vi "Error Bar Page.vi"() -> ()   [LabVIEW 2017, in "2D Error Bar.lvclass"]
uses:
  <vilib>/Math Plots/2D Math Plots/2D Error Bar/2D Error Bar/2D Error Bar.lvclass
  <vilib>/Math Plots/2D Math Plots/2D Plot/Action String/2DMathPlot Ctrl Act Queue.ctl
  <vilib>/Math Plots/2D Math Plots/2D Plot/Action String/2DMathPlot Ctrl Act Cluster.ctl
  <vilib>/Math Plots/2D Math Plots/2D Plot/Action String/2DMathPlot State Class.ctl
  <vilib>/Math Plots/2D Math Plots/2D Error Bar/2D Error Bar/Typedef/2D Error Bar Property Cluster.ctl
  <vilib>/Math Plots/2D Math Plots/2D Plot/2D Plot/Typedef/Plot Property Array.ctl
  <vilib>/Math Plots/2D Math Plots/2D Plot/2D Plot/Typedef/Plot Property.ctl
  <vilib>/Math Plots/2D Math Plots/2D Error Bar/2D Error Bar/Typedef/2D Error Bar Property Array.ctl
  <vilib>/Math Plots/2D Math Plots/2D Error Bar/2D Error Bar/Typedef/2D Error Bar Property.ctl
  <vilib>/Math Plots/2D Math Plots/2D Plot/2D Plot/Typedef/Dialog State.ctl
  <vilib>/Math Plots/2D Math Plots/2D Plot/2D Plot/Typedef/Temp Graph State.ctl
  <vilib>/Math Plots/2D Math Plots/2D Plot/2D Plot/Typedef/Temp Graph Property Action.ctl
  <vilib>/Math Plots/2D Math Plots/2D Plot/2D Plot/2D Plot.lvclass
panel:
  in  "Fill to":i32(ring)=-1 items=["<none>"=-1, "zero"=-2, "-Infinity"=-3, "+Infinity"=-4, "-"=100]
  in  "Errorbar Point/fill":u32(colorbox)=16777215 caption="Point/fill color"
  in  "Errorbar Interpolation":T1
  in  "Errorbar Line Width":T2
  in  "Errorbar Point Style":T3
  in  "Errorbar Line Style":T4
  in  "Errorbar Line Color":u32(colorbox) caption="Line color"
  in  "Error Mode":u16(ring) items=["Y errorbar", "XY errorbar"]
  in  "Marker Color":u32(colorbox) caption="Marker color"
  out "Error Bar Property Out":T5={"Plot Property Array"=[{"Bar Plot Style"=0, "DigitalLineStyle"=1, "TransitionLocation"=0, "Transition Type"=0, "Fill To"=0, "Fill/Pt. Color"=0, "Label Style"=0, "Line Style"=0, "Line Width"=0, "Plot Color"=0, "Plot Interpolation"=0, "Plot Name"="", "Point Style"=0, "Visible?"=FALSE, "XScaleIdx"=0, "YScaleIdx"=0}, {"Bar Plot Style"=0, "DigitalLineStyle"=1, "TransitionLocation"=0, "Transition Type"=0, "Fill To"=0, "Fill/Pt. Color"=0, "Label Style"=0, "Line Style"=0, "Line Width"=0, "Plot Color"=0, "Plot Interpolation"=0, "Plot Name"="", "Point Style"=0, "Visible?"=FALSE, "XScaleIdx"=0, "YScaleIdx"=0}], "2D Error Bar Property Array"=[]}
  in  "Error Bar Property In":T5={"Plot Property Array"=[{"Bar Plot Style"=0, "DigitalLineStyle"=1, "TransitionLocation"=0, "Transition Type"=0, "Fill To"=0, "Fill/Pt. Color"=0, "Label Style"=0, "Line Style"=0, "Line Width"=0, "Plot Color"=0, "Plot Interpolation"=0, "Plot Name"="", "Point Style"=0, "Visible?"=FALSE, "XScaleIdx"=0, "YScaleIdx"=0}, {"Bar Plot Style"=0, "DigitalLineStyle"=1, "TransitionLocation"=0, "Transition Type"=0, "Fill To"=0, "Fill/Pt. Color"=0, "Label Style"=0, "Line Style"=0, "Line Width"=0, "Plot Color"=0, "Plot Interpolation"=0, "Plot Name"="", "Point Style"=0, "Visible?"=FALSE, "XScaleIdx"=0, "YScaleIdx"=0}], "2D Error Bar Property Array"=[]}
  in  "Event Registration":refnum<event-registration>
  in  "Control Ref Queue":T10
  in  "Marker Size":dbl=0.001 caption="Size" min=0.001 step=1.0
  in  "Marker Line Width":T2
  in  "Marker Line Style":T4
  in  "Name":string
  in  "Active Plot":i32(ring) items=["Plot 0"]
  # "Error Bar"
  # "Error Marker"
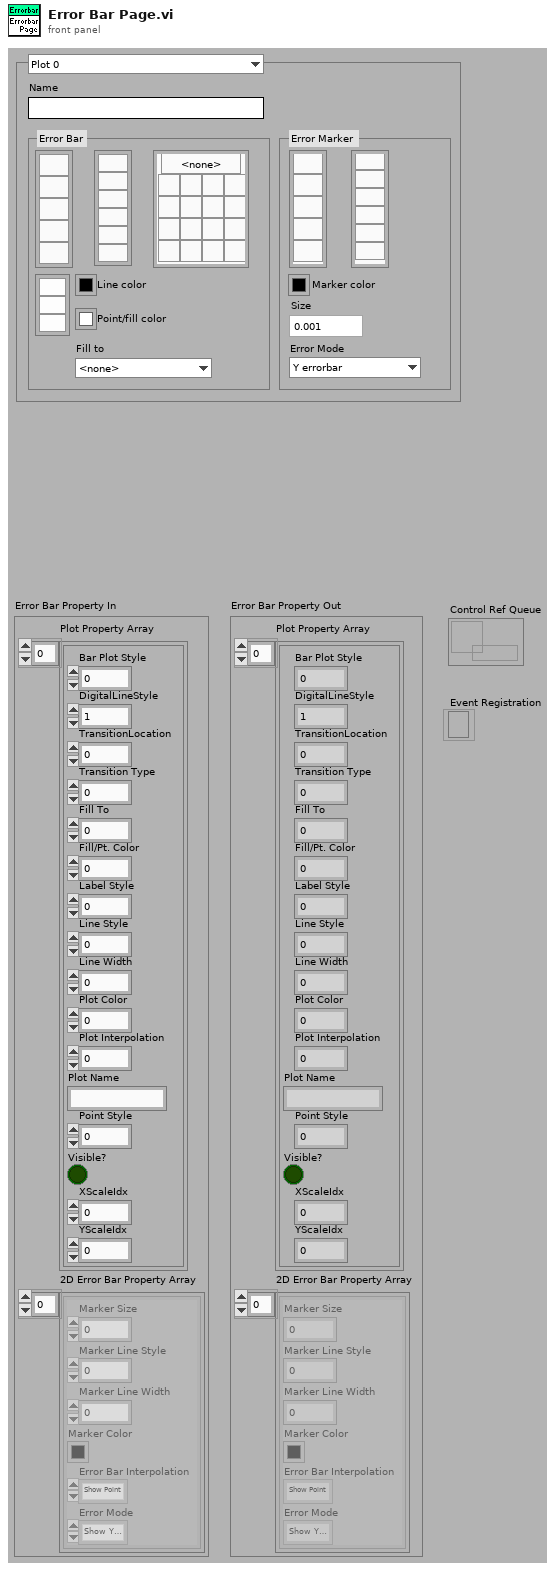
[diagram p1: front panel]
types:
  T1 = cluster{"OK Button 2":bool, "OK Button 4":bool, "OK Button 6":bool}
  T2 = cluster{"OK Button 2":bool, "OK Button 3":bool, "OK Button 4":bool, "OK Button 5":bool, "OK Button 6":bool, "OK Button 7":bool}
  T3 = cluster{"OK Button 17":bool, "OK Button":bool, "OK Button 2":bool, "OK Button 3":bool, "OK Button 4":bool, "OK Button 5":bool, "OK Button 6":bool, "OK Button 7":bool, "OK Button 8":bool, "OK Button 9":bool, "OK Button 10":bool, "OK Button 11":bool, "OK Button 12":bool, "OK Button 13":bool, "OK Button 14":bool, "OK Button 15":bool, "OK Button 16":bool}
  T4 = cluster{"OK Button":bool, "OK Button 2":bool, "OK Button 3":bool, "OK Button 4":bool, "OK Button 5":bool}
  T5 = typedef "2D Error Bar.lvclass/2D Error Bar Property Cluster.ctl" = cluster{"Plot Property Array":T6, "2D Error Bar Property Array":T8}
  T6 = typedef "2D Plot.lvclass/Plot Property Array.ctl" = T7[]
  T7 = typedef "2D Plot.lvclass/Plot Property.ctl" = cluster{"Bar Plot Style":u8, "DigitalLineStyle":u8, "TransitionLocation":u8, "Transition Type":u8, "Fill To":i16, "Fill/Pt. Color":u32, "Label Style":u8, "Line Style":u8, "Line Width":u8, "Plot Color":u32, "Plot Interpolation":u8, "Plot Name":string, "Point Style":u8, "Visible?":bool, "XScaleIdx":u32, "YScaleIdx":u32}
  T8 = typedef "2D Error Bar.lvclass/2D Error Bar Property Array.ctl" = T9[]
  T9 = typedef "2D Error Bar.lvclass/2D Error Bar Property.ctl" = cluster{"Marker Size":dbl, "Marker Line Style":u8, "Marker Line Width":u8, "Marker Color":u32, "Error Bar Interpolation":enum16{"Show Point", "Show Line", "Show Bar"}, "Error Mode":enum16{"Show Y Error", "Show X Error", "Show Both Error"}}
  T10 = typedef "2DMathPlot Ctrl Act Queue.ctl" = refnum<queue>
  T11 = typedef "2D Plot.lvclass/Dialog State.ctl" = enum16{"Initialize", "Read Property", "Write Property", "Idle", "Exit"}
  T12 = typedef "2DMathPlot Ctrl Act Cluster.ctl" = cluster{"Plot Area Ref":refnum<vi>, "Z Axis Ref":refnum<vi>, "Legend Ref":refnum<vi>, "XControl Ref":refnum<vi>, "Facade Ref":refnum<vi>, "Display State Change Class":T13}
  T13 = typedef "2DMathPlot State Class.ctl" = enum16{"Update All (Undo)", "Update General", "Update Appearance", "Update Format", "Update Scale", "Update Marker", "Update Cursor", "None"}
  T14 = typedef "2D Plot.lvclass/Temp Graph Property Action.ctl" = enum16{"Appearance Property", "Format Property", "Plots Property", "Scales Property"}
  T15 = typedef "2D Plot.lvclass/Temp Graph State.ctl" = enum16{"Create", "Update Graph", "Update Property Only", "Get Plot Name", "Get Axis Name", "Destory"}
  T16 = enum16{"Show Y Error", "Show X Error", "Show Both Error"}
  T17 = cluster{"Bool Array[0]":bool, "Bool Array[1]":bool, "Bool Array[2]":bool, "Bool Array[3]":bool, "Bool Array[4]":bool}
  T18 = cluster{"Bool Array[0]":bool, "Bool Array[1]":bool, "Bool Array[2]":bool, "Bool Array[3]":bool, "Bool Array[4]":bool, "Bool Array[5]":bool}
  T19 = cluster{"Bool Array[0]":bool, "Bool Array[1]":bool, "Bool Array[2]":bool, "Bool Array[3]":bool, "Bool Array[4]":bool, "Bool Array[5]":bool, "Bool Array[6]":bool, "Bool Array[7]":bool, "Bool Array[8]":bool, "Bool Array[9]":bool, "Bool Array[10]":bool, "Bool Array[11]":bool, "Bool Array[12]":bool, "Bool Array[13]":bool, "Bool Array[14]":bool, "Bool Array[15]":bool, "Bool Array[16]":bool}
  T20 = cluster{"Bool Array[0]":bool, "Bool Array[1]":bool, "Bool Array[2]":bool}
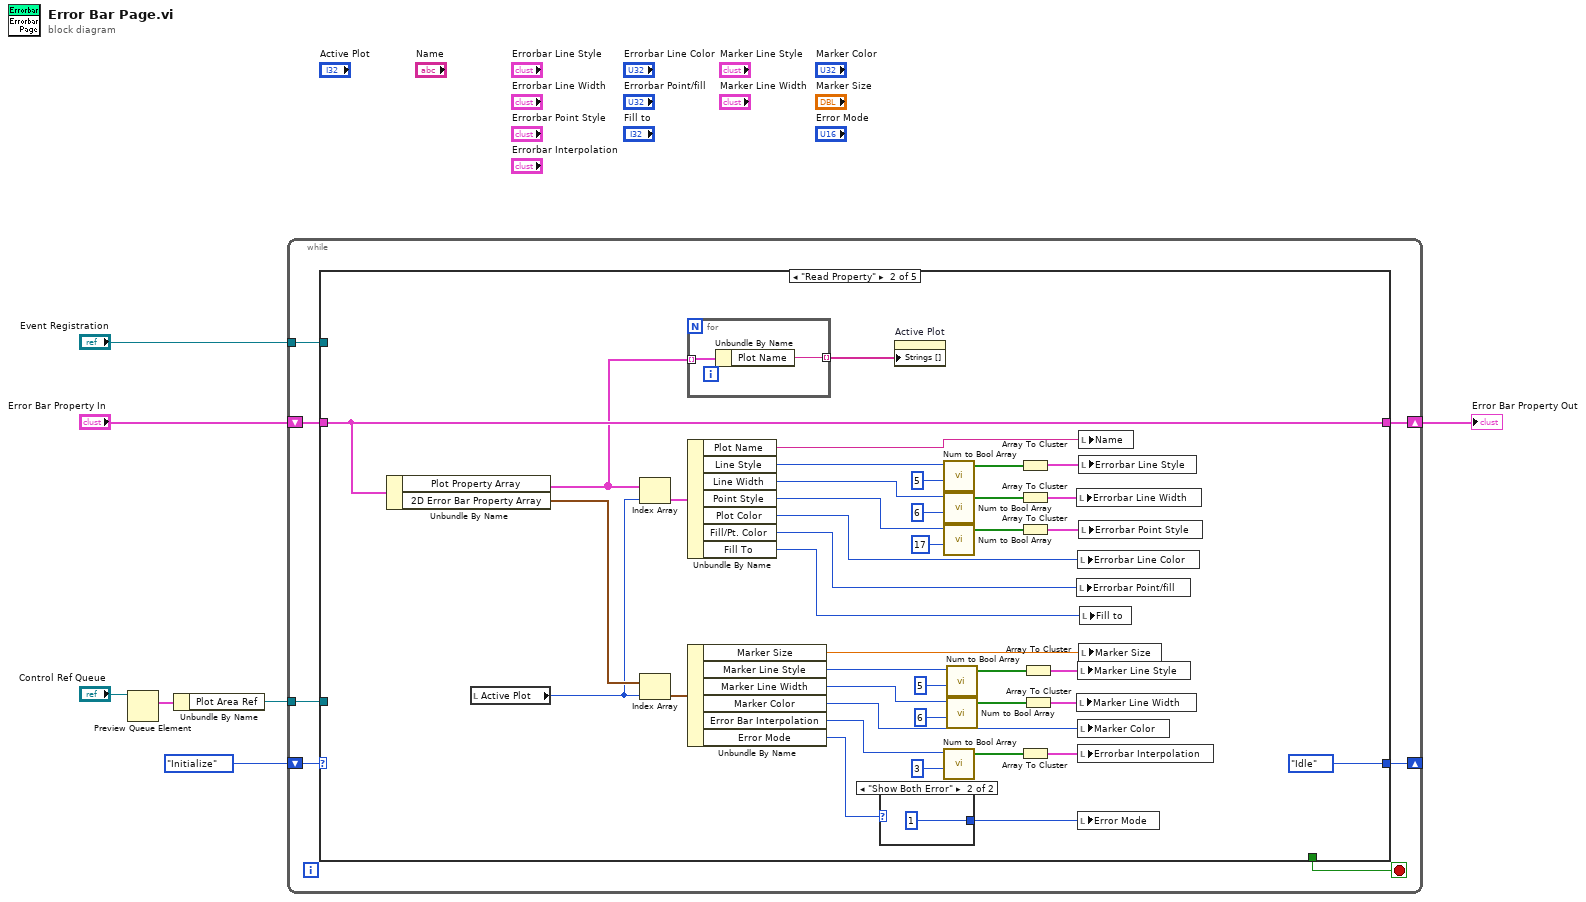
[diagram p0: block diagram]
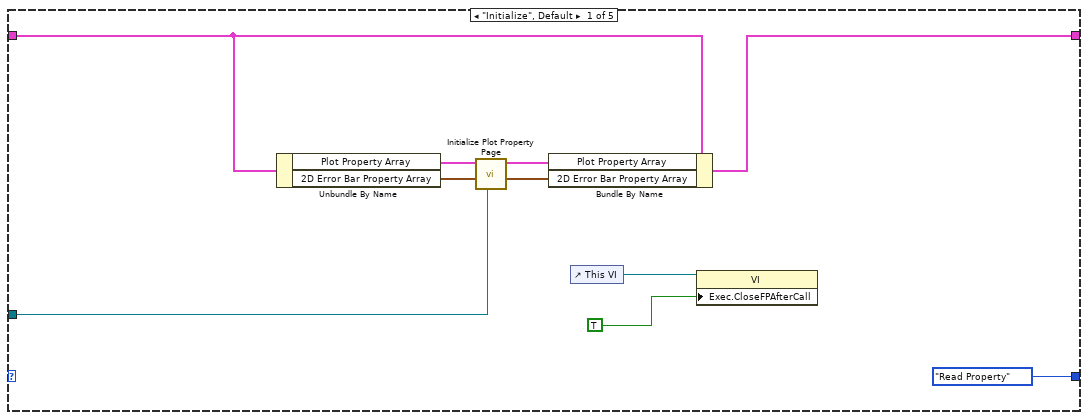
[diagram p2: hidden frame]
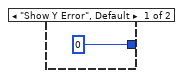
[diagram p3: hidden frame]
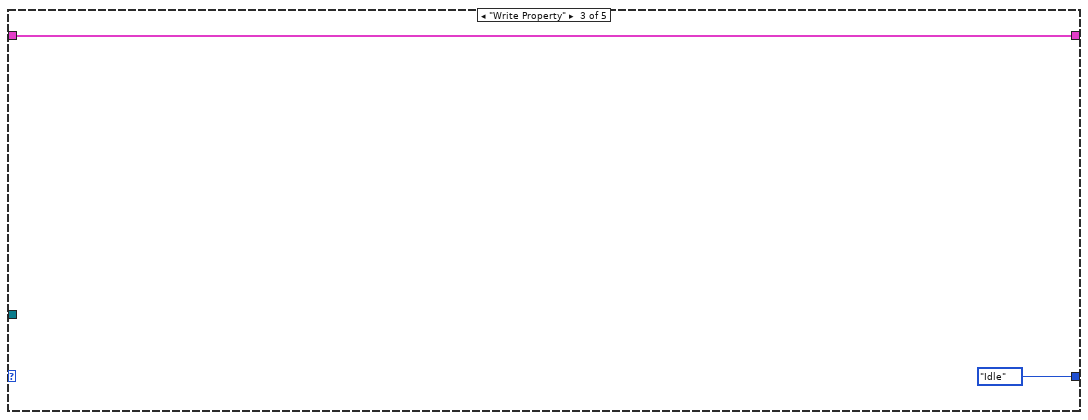
[diagram p4: hidden frame]
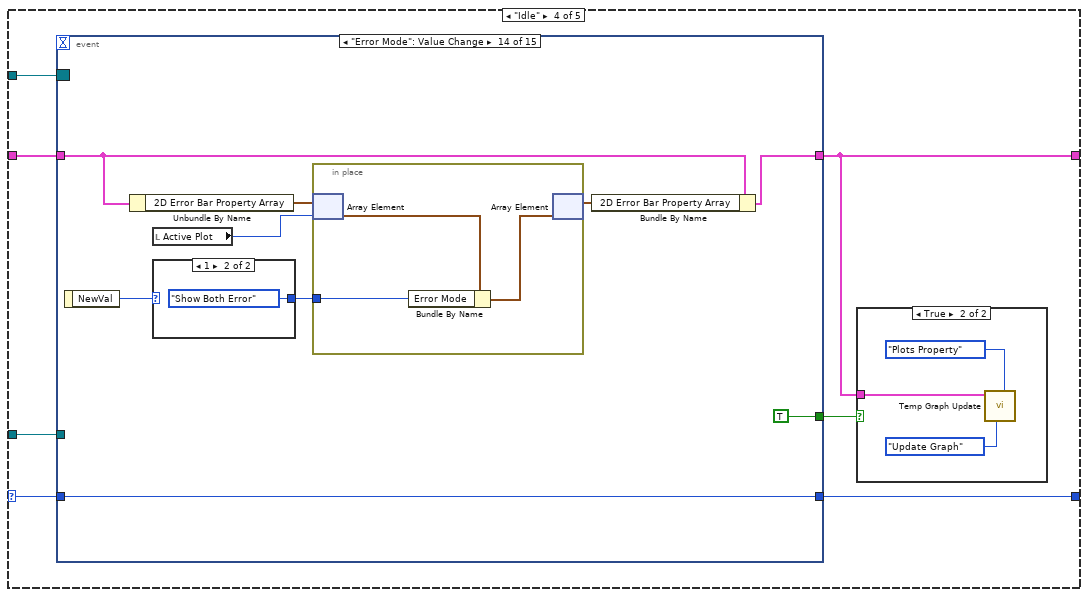
[diagram p5: hidden frame]
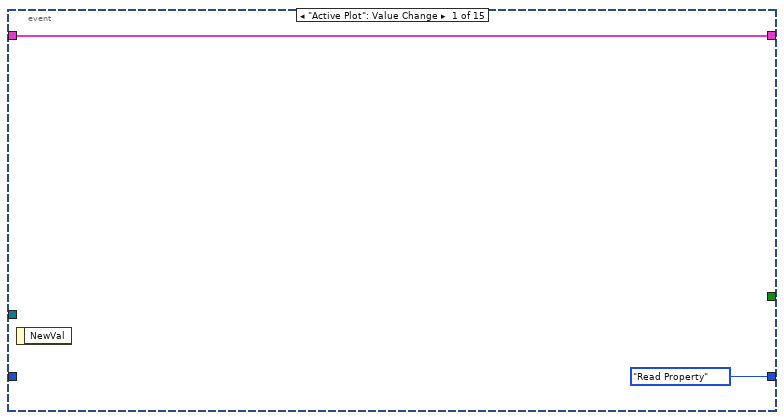
[diagram p7: hidden frame]
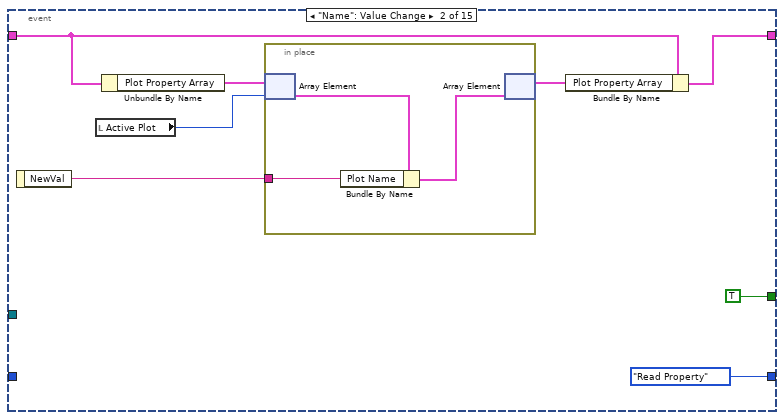
[diagram p8: hidden frame]
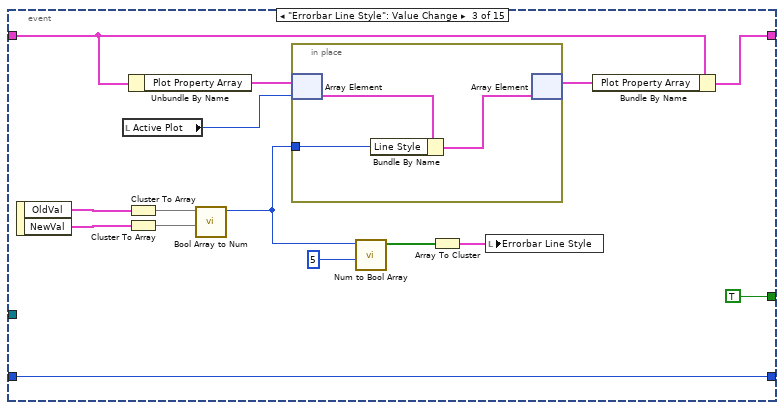
[diagram p9: hidden frame]
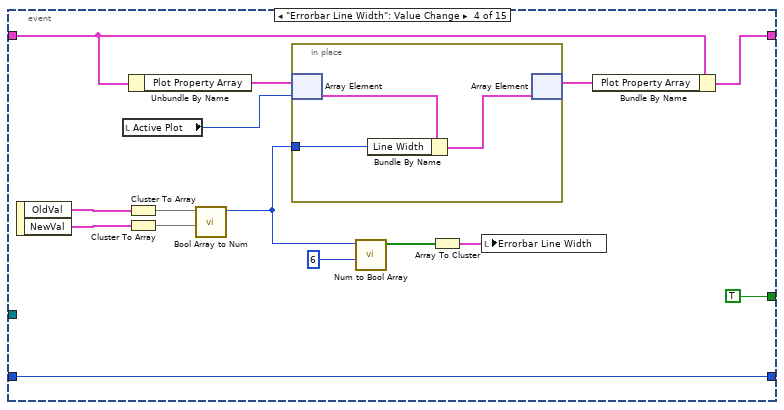
[diagram p10: hidden frame]
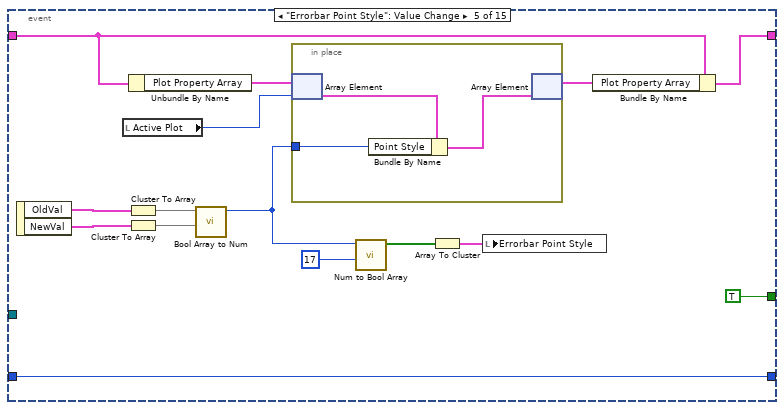
[diagram p11: hidden frame]
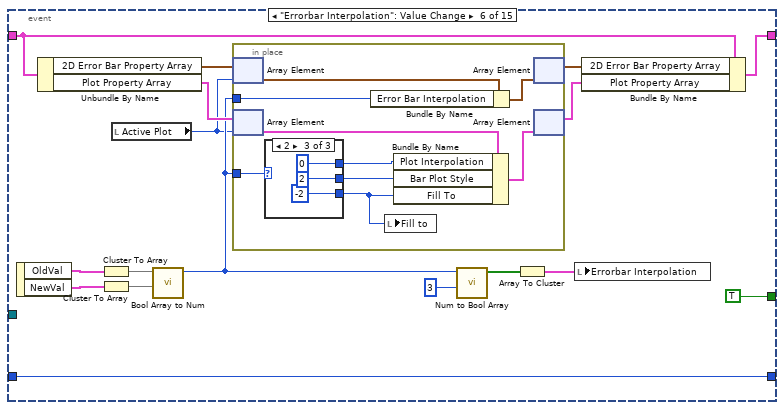
[diagram p12: hidden frame]
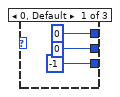
[diagram p13: hidden frame]
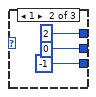
[diagram p14: hidden frame]
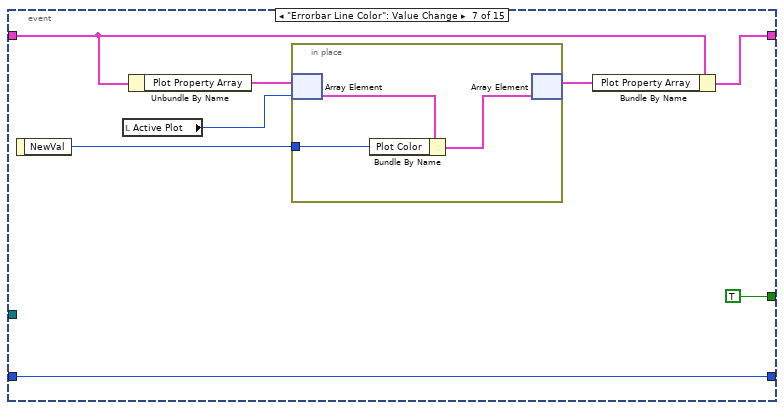
[diagram p15: hidden frame]
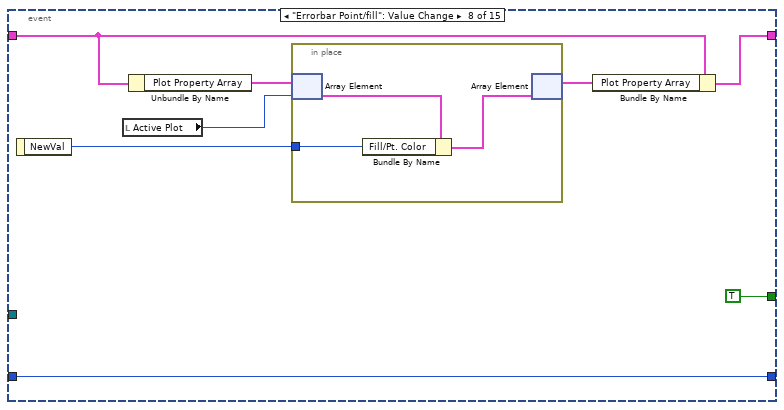
[diagram p16: hidden frame]
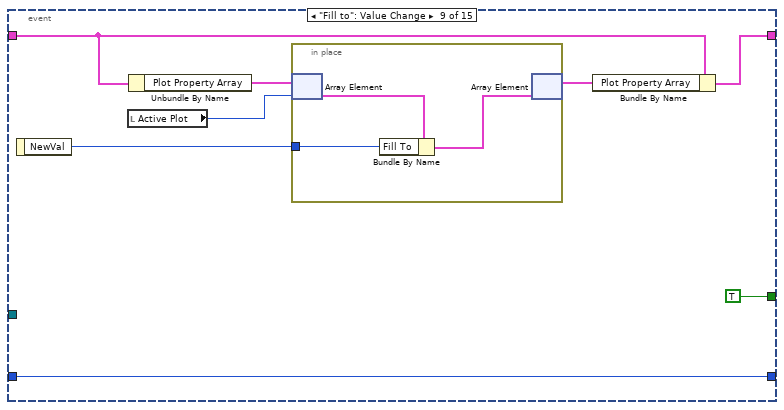
[diagram p17: hidden frame]
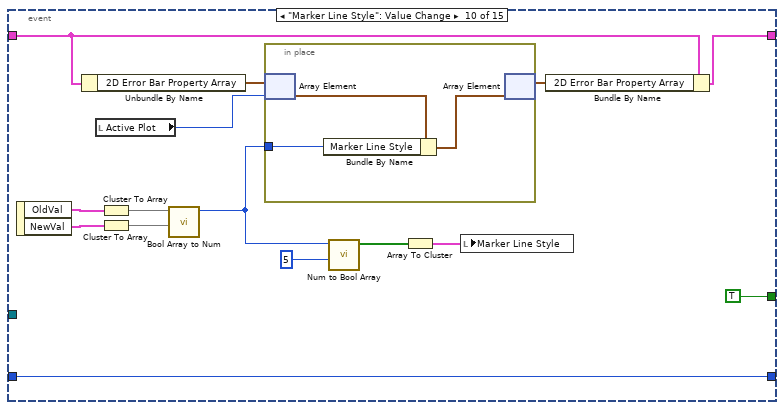
[diagram p18: hidden frame]
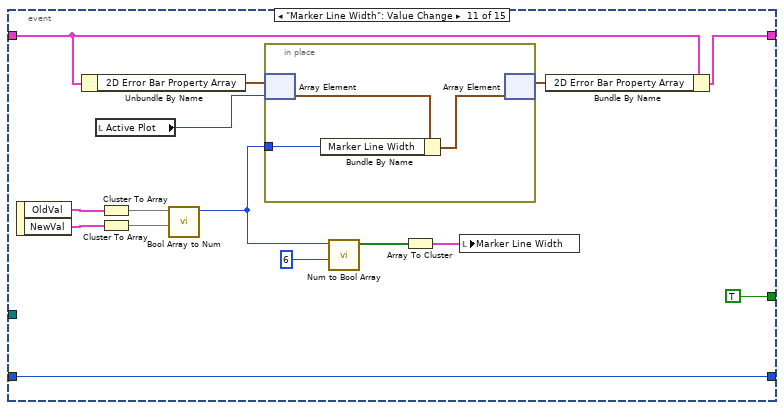
[diagram p19: hidden frame]
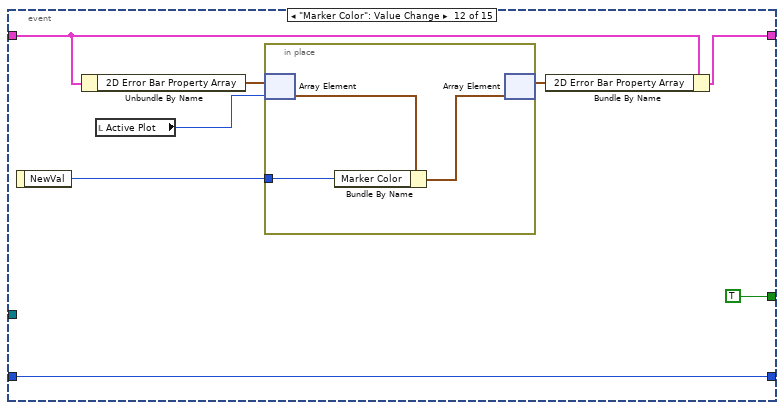
[diagram p20: hidden frame]
diagram:
  n1 = Preview Queue Element(queue="Control Ref Queue") -> (element=w5:T12)  [unwired: 1 in, 4 out]
  n2 = Unbundle By Name(w5) -> ("Plot Area Ref"=w4:refnum<vi>)
  n3 = while {
    tunnel: w4 -> [w13]
    tunnel: "Event Registration" -> [w12]
    shift-right: [w9] -> _
    shift-left: Dialog_State."Initialize" ("Enum") -> [w14]
    shift-right: [w10] -> w1
    shift-left: "Error Bar Property In" -> [w11]
    stop <- w8 stop-if-true
    n4 = case shown="\"Read Property\"" w14 {
      selector: w14 -> [_ _ _ w74 w292]
      tunnel: w13 -> [w15 _ _ w75 _]
      tunnel: w12 -> [_ _ _ w77 _]
      tunnel: w11 -> [w21 w61 w69 w76 w290]
      tunnel: [w20 w61 w69 w73 w290] -> w10
      tunnel: [Dialog_State."Read Property" ("Enum") Dialog_State."Idle" ("Enum") Dialog_State."Idle" ("Enum") w72 w292] -> w9
      tunnel: [_ _ _ _ TRUE] -> w8
      frame "Initialize", Default {
        n5 = Unbundle By Name(w21) -> ("Plot Property Array"=w19:T6, "2D Error Bar Property Array"=w18:T8)
        n6 = call <vilib>:"Initialize Plot Property Page.vi"("Plot Area Ref"=w15, "2D Error Bar Array In"=w18, "Plot Property Array In"=w19) -> ("2D Error Bar Array Out"=w16:T8, "Plot Property Array Out"=w17:T6)  [unwired: 2 in, 5 out]
        n7 = Bundle By Name(cluster=w21, "Plot Property Array"=w17, "2D Error Bar Property Array"=w16) -> (w20:T5)
        n8 = control-ref of="This VI"() -> (w23:refnum<vi>)
        n9 = property class="VI"(reference=w23, "Exec.CloseFPAfterCall"=TRUE ("Execution:Close After Call")) -> ()  [unwired: 1 in, 2 out]
      }
      frame "Read Property" {
        n10 = Unbundle By Name(w61) -> ("Plot Property Array"=w49:T6, "2D Error Bar Property Array"=w64:T8)
        n11 = local read "Active Plot"() -> (w28:i32)
        n12 = Index Array(array=w49, index=w28) -> (element=w63:T7)
        n13 = Index Array(array=w64, index=w28) -> (element=w62:T9)
        n14 = for {
          tunnel: w49 -> [w68] mode=indexing
          tunnel: [w67] -> w48 mode=indexing
          n15 = Unbundle By Name(w68) -> ("Plot Name"=w67:string)
        }
        n16 = Unbundle By Name(w63) -> ("Plot Name"=w59:string, "Line Style"=w58:u8, "Line Width"=w51:u8, "Point Style"=w35:u8, "Plot Color"=w32:u32, "Fill/Pt. Color"=w31:u32, "Fill To"=w30:i16)
        n17 = Unbundle By Name(w62) -> ("Marker Size"=w60:dbl, "Marker Line Style"=w43:u8, "Marker Line Width"=w41:u8, "Marker Color"=w25:u32, "Error Bar Interpolation"=w29:enum16{"Show Point", "Show Line", "Show Bar"}, "Error Mode"=w27:T16)
        n18 = case shown="\"Show Both Error\"" w27 {
          tunnel: [0 1] -> w26
          frame "Show Y Error", Default {
          }
          frame "Show Both Error" {
          }
        }
        n19 = property on="Active Plot" class="Ring (strict)"("Strings []"=w48) -> ()  [unwired: 2 in, 2 out]
        n20 = call <vilib>:"Num to Bool Array.vi"("Array Size"=5, "Value"=w58) -> ("Bool Array"=w56:bool[])  [unwired: 9 out]
        n21 = call <vilib>:"Num to Bool Array.vi"("Array Size"=6, "Value"=w51) -> ("Bool Array"=w54:bool[])  [unwired: 9 out]
        n22 = call <vilib>:"Num to Bool Array.vi"("Array Size"=17, "Value"=w35) -> ("Bool Array"=w37:bool[])  [unwired: 9 out]
        n23 = call <vilib>:"Num to Bool Array.vi"("Array Size"=3, "Value"=w29) -> ("Bool Array"=w39:bool[])  [unwired: 9 out]
        n24 = call <vilib>:"Num to Bool Array.vi"("Array Size"=5, "Value"=w43) -> ("Bool Array"=w45:bool[])  [unwired: 9 out]
        n25 = call <vilib>:"Num to Bool Array.vi"("Array Size"=6, "Value"=w41) -> ("Bool Array"=w46:bool[])  [unwired: 9 out]
        n26 = Array To Cluster(array=w56) -> (cluster=w55:T17)
        n27 = Array To Cluster(array=w54) -> (cluster=w52:T18)
        n28 = Array To Cluster(array=w37) -> (cluster=w33:T19)
        n29 = Array To Cluster(array=w39) -> (cluster=w34:T20)
        n30 = Array To Cluster(array=w45) -> (cluster=w42:T17)
        n31 = Array To Cluster(array=w46) -> (cluster=w40:T18)
        n32 = local write "Errorbar Line Width"(w52) -> ()
        n33 = local write "Errorbar Point/fill"(w31) -> ()
        n34 = local write "Marker Line Width"(w40) -> ()
        n35 = local write "Errorbar Line Color"(w32) -> ()
        n36 = local write "Marker Line Style"(w42) -> ()
        n37 = local write "Marker Color"(w25) -> ()
        n38 = local write "Errorbar Interpolation"(w34) -> ()
        n39 = local write "Error Mode"(w26) -> ()
        n40 = local write "Name"(w59) -> ()
        n41 = local write "Errorbar Line Style"(w55) -> ()
        n42 = local write "Errorbar Point Style"(w33) -> ()
        n43 = local write "Marker Size"(w60) -> ()
        n44 = local write "Fill to"(w30) -> ()
      }
      frame "Write Property" {
      }
      frame "Idle" {
        n45 = event shown="[13] \"Error Mode\": Value Change" {
          selector: w77 -> [_ _ _ _ _ _ _ _ _ _ _ _ _ _ _]
          dyn-events: _ -> [_ _ _ _ _ _ _ _ _ _ _ _ _ _ _]
          timeout: _ -> [_ _ _ _ _ _ _ _ _ _ _ _ _ _ _]
          tunnel: w76 -> [w82 w90 w100 w118 w136 w157 w187 w198 w209 w230 w248 w259 w270 w282 w288]
          tunnel: w75 -> [_ _ _ _ _ _ _ _ _ _ _ _ _ _ _]
          tunnel: [w82 w89 w99 w117 w135 w156 w186 w197 w208 w229 w247 w258 w269 w281 w288] -> w73
          tunnel: [Dialog_State."Read Property" ("Enum") Dialog_State."Read Property" ("Enum") w96 w114 w132 w153 w185 w196 w207 w218 w235 w254 w265 w277 Dialog_State."Exit" ("Enum")] -> w72
          tunnel: w74 -> [_ _ w96 w114 w132 w153 w185 w196 w207 w218 w235 w254 w265 w277 _]
          tunnel: [_ TRUE TRUE TRUE TRUE TRUE TRUE TRUE TRUE TRUE TRUE TRUE TRUE TRUE _] -> w71
          event "Active Plot": Value Change {
            n46 = event-data() -> ()  [unwired: 2 out]
          }
          event "Name": Value Change {
            n47 = event-data() -> ("NewVal"=w85:string)  [unwired: 1 out]
            n48 = local read "Active Plot"() -> (w87:i32)
            n49 = Unbundle By Name(w90) -> ("Plot Property Array"=w88:T6)
            n50 = in-place {
              in-place-border: w85 -> [w91]
              n51 = in-place-array #1(w88, w87) -> (w93:T7)
              n52 = Bundle By Name(cluster=w93, "Plot Name"=w91) -> (w92:T7)
              n53 = in-place-array #1(w92) -> (w86:T6)  [unwired: 1 out]
            }
            n54 = Bundle By Name(cluster=w90, "Plot Property Array"=w86) -> (w89:T5)
          }
          event "Errorbar Line Style": Value Change {
            n55 = event-data() -> ("OldVal"=w98:T4, "NewVal"=w97:T4)  [unwired: 1 out]
            n56 = local read "Active Plot"() -> (w101:i32)
            n57 = Cluster To Array(cluster=w98) -> (array=w104:bool[])
            n58 = Cluster To Array(cluster=w97) -> (array=w103:bool[])
            n59 = Unbundle By Name(w100) -> ("Plot Property Array"=w108:T6)
            n60 = call <vilib>:"Bool Array to Num.vi"("New Bool Array"=w103, "Old Bool Array"=w104) -> ("Value"=w95:u8)  [unwired: 9 out]
            n61 = in-place {
              in-place-border: w95 -> [w109]
              n62 = in-place-array #2(w108, w101) -> (w111:T7)
              n63 = Bundle By Name(cluster=w111, "Line Style"=w109) -> (w110:T7)
              n64 = in-place-array #2(w110) -> (w107:T6)  [unwired: 1 out]
            }
            n65 = call <vilib>:"Num to Bool Array.vi"("Array Size"=5, "Value"=w95) -> ("Bool Array"=w106:bool[])  [unwired: 9 out]
            n66 = Array To Cluster(array=w106) -> (cluster=w102:T17)
            n67 = local write "Errorbar Line Style"(w102) -> ()
            n68 = Bundle By Name(cluster=w100, "Plot Property Array"=w107) -> (w99:T5)
          }
          event "Errorbar Line Width": Value Change {
            n69 = event-data() -> ("OldVal"=w116:T2, "NewVal"=w115:T2)  [unwired: 1 out]
            n70 = local read "Active Plot"() -> (w119:i32)
            n71 = Cluster To Array(cluster=w116) -> (array=w122:bool[])
            n72 = Cluster To Array(cluster=w115) -> (array=w121:bool[])
            n73 = Unbundle By Name(w118) -> ("Plot Property Array"=w126:T6)
            n74 = call <vilib>:"Bool Array to Num.vi"("New Bool Array"=w121, "Old Bool Array"=w122) -> ("Value"=w113:u8)  [unwired: 9 out]
            n75 = in-place {
              in-place-border: w113 -> [w127]
              n76 = in-place-array #3(w126, w119) -> (w129:T7)
              n77 = Bundle By Name(cluster=w129, "Line Width"=w127) -> (w128:T7)
              n78 = in-place-array #3(w128) -> (w125:T6)  [unwired: 1 out]
            }
            n79 = call <vilib>:"Num to Bool Array.vi"("Array Size"=6, "Value"=w113) -> ("Bool Array"=w124:bool[])  [unwired: 9 out]
            n80 = Array To Cluster(array=w124) -> (cluster=w120:T18)
            n81 = local write "Errorbar Line Width"(w120) -> ()
            n82 = Bundle By Name(cluster=w118, "Plot Property Array"=w125) -> (w117:T5)
          }
          event "Errorbar Point Style": Value Change {
            n83 = event-data() -> ("OldVal"=w134:T3, "NewVal"=w133:T3)  [unwired: 1 out]
            n84 = local read "Active Plot"() -> (w137:i32)
            n85 = Cluster To Array(cluster=w134) -> (array=w140:bool[])
            n86 = Cluster To Array(cluster=w133) -> (array=w139:bool[])
            n87 = Unbundle By Name(w136) -> ("Plot Property Array"=w144:T6)
            n88 = call <vilib>:"Bool Array to Num.vi"("New Bool Array"=w139, "Old Bool Array"=w140) -> ("Value"=w131:u8)  [unwired: 9 out]
            n89 = in-place {
              in-place-border: w131 -> [w145]
              n90 = in-place-array #4(w144, w137) -> (w147:T7)
              n91 = Bundle By Name(cluster=w147, "Point Style"=w145) -> (w146:T7)
              n92 = in-place-array #4(w146) -> (w143:T6)  [unwired: 1 out]
            }
            n93 = call <vilib>:"Num to Bool Array.vi"("Array Size"=17, "Value"=w131) -> ("Bool Array"=w142:bool[])  [unwired: 9 out]
            n94 = Array To Cluster(array=w142) -> (cluster=w138:T19)
            n95 = local write "Errorbar Point Style"(w138) -> ()
            n96 = Bundle By Name(cluster=w136, "Plot Property Array"=w143) -> (w135:T5)
          }
          event "Errorbar Interpolation": Value Change {
            n97 = event-data() -> ("OldVal"=w155:T1, "NewVal"=w154:T1)  [unwired: 1 out]
            n98 = Unbundle By Name(w157) -> ("2D Error Bar Property Array"=w151:T8, "Plot Property Array"=w164:T6)
            n99 = Cluster To Array(cluster=w155) -> (array=w160:bool[])
            n100 = Cluster To Array(cluster=w154) -> (array=w159:bool[])
            n101 = local read "Active Plot"() -> (w149:i32)
            n102 = call <vilib>:"Bool Array to Num.vi"("New Bool Array"=w159, "Old Bool Array"=w160) -> ("Value"=w152:u8)  [unwired: 9 out]
            n103 = in-place {
              in-place-border: w152 -> [w169]
              in-place-border: w152 -> [w168]
              n104 = in-place-array #5(w151, w149) -> (w171:T9)
              n105 = in-place-array #6(w164, w149) -> (w173:T7)
              n106 = case shown="2" w168 {
                tunnel: [u8 0 ("Plot Interpolation") u8 2 ("Plot Interpolation") u8 0 ("Plot Interpolation")] -> w167
                tunnel: [u8 0 ("Plot Interpolation") u8 0 ("Plot Interpolation") u8 2 ("Plot Interpolation")] -> w166
                tunnel: [i16 -1 ("Fill To") i16 -1 ("Fill To") i16 -2 ("Fill To")] -> w165
                frame 0, Default {
                }
                frame 1 {
                }
                frame 2 {
                }
              }
              n107 = Bundle By Name(cluster=w171, "Error Bar Interpolation"=w169) -> (w170:T9)
              n108 = local write "Fill to"(w165) -> ()
              n109 = Bundle By Name(cluster=w173, "Plot Interpolation"=w167, "Bar Plot Style"=w166, "Fill To"=w165) -> (w172:T7)
              n110 = in-place-array #5(w170) -> (w150:T8)  [unwired: 1 out]
              n111 = in-place-array #6(w172) -> (w163:T6)  [unwired: 1 out]
            }
            n112 = call <vilib>:"Num to Bool Array.vi"("Array Size"=3, "Value"=w152) -> ("Bool Array"=w162:bool[])  [unwired: 9 out]
            n113 = Array To Cluster(array=w162) -> (cluster=w158:T20)
            n114 = local write "Errorbar Interpolation"(w158) -> ()
            n115 = Bundle By Name(cluster=w157, "2D Error Bar Property Array"=w150, "Plot Property Array"=w163) -> (w156:T5)
          }
          event "Errorbar Line Color": Value Change {
            n116 = event-data() -> ("NewVal"=w184:u32)  [unwired: 1 out]
            n117 = local read "Active Plot"() -> (w188:i32)
            n118 = Unbundle By Name(w187) -> ("Plot Property Array"=w190:T6)
            n119 = in-place {
              in-place-border: w184 -> [w191]
              n120 = in-place-array #7(w190, w188) -> (w193:T7)
              n121 = Bundle By Name(cluster=w193, "Plot Color"=w191) -> (w192:T7)
              n122 = in-place-array #7(w192) -> (w189:T6)  [unwired: 1 out]
            }
            n123 = Bundle By Name(cluster=w187, "Plot Property Array"=w189) -> (w186:T5)
          }
          event "Errorbar Point/fill": Value Change {
            n124 = event-data() -> ("NewVal"=w195:u32)  [unwired: 1 out]
            n125 = local read "Active Plot"() -> (w199:i32)
            n126 = Unbundle By Name(w198) -> ("Plot Property Array"=w201:T6)
            n127 = in-place {
              in-place-border: w195 -> [w202]
              n128 = in-place-array #8(w201, w199) -> (w204:T7)
              n129 = Bundle By Name(cluster=w204, "Fill/Pt. Color"=w202) -> (w203:T7)
              n130 = in-place-array #8(w203) -> (w200:T6)  [unwired: 1 out]
            }
            n131 = Bundle By Name(cluster=w198, "Plot Property Array"=w200) -> (w197:T5)
          }
          event "Fill to": Value Change {
            n132 = event-data() -> ("NewVal"=w206:i32)  [unwired: 1 out]
            n133 = local read "Active Plot"() -> (w210:i32)
            n134 = Unbundle By Name(w209) -> ("Plot Property Array"=w212:T6)
            n135 = in-place {
              in-place-border: w206 -> [w213]
              n136 = in-place-array #9(w212, w210) -> (w215:T7)
              n137 = Bundle By Name(cluster=w215, "Fill To"=w213) -> (w214:T7)
              n138 = in-place-array #9(w214) -> (w211:T6)  [unwired: 1 out]
            }
            n139 = Bundle By Name(cluster=w209, "Plot Property Array"=w211) -> (w208:T5)
          }
          event "Marker Line Style": Value Change {
            n140 = event-data() -> ("OldVal"=w222:T4, "NewVal"=w221:T4)  [unwired: 1 out]
            n141 = Unbundle By Name(w230) -> ("2D Error Bar Property Array"=w228:T8)
            n142 = local read "Active Plot"() -> (w217:i32)
            n143 = Cluster To Array(cluster=w222) -> (array=w224:bool[])
            n144 = Cluster To Array(cluster=w221) -> (array=w223:bool[])
            n145 = call <vilib>:"Bool Array to Num.vi"("New Bool Array"=w223, "Old Bool Array"=w224) -> ("Value"=w219:u8)  [unwired: 9 out]
            n146 = in-place {
              in-place-border: w219 -> [w231]
              n147 = in-place-array #10(w228, w217) -> (w233:T9)
              n148 = Bundle By Name(cluster=w233, "Marker Line Style"=w231) -> (w232:T9)
              n149 = in-place-array #10(w232) -> (w227:T8)  [unwired: 1 out]
            }
            n150 = call <vilib>:"Num to Bool Array.vi"("Array Size"=5, "Value"=w219) -> ("Bool Array"=w226:bool[])  [unwired: 9 out]
            n151 = Array To Cluster(array=w226) -> (cluster=w220:T17)
            n152 = local write "Marker Line Style"(w220) -> ()
            n153 = Bundle By Name(cluster=w230, "2D Error Bar Property Array"=w227) -> (w229:T5)
          }
          event "Marker Line Width": Value Change {
            n154 = event-data() -> ("OldVal"=w239:T2, "NewVal"=w238:T2)  [unwired: 1 out]
            n155 = Unbundle By Name(w248) -> ("2D Error Bar Property Array"=w246:T8)
            n156 = local read "Active Plot"() -> (w245:i32)
            n157 = Cluster To Array(cluster=w239) -> (array=w241:bool[])
            n158 = Cluster To Array(cluster=w238) -> (array=w240:bool[])
            n159 = call <vilib>:"Bool Array to Num.vi"("New Bool Array"=w240, "Old Bool Array"=w241) -> ("Value"=w236:u8)  [unwired: 9 out]
            n160 = in-place {
              in-place-border: w236 -> [w249]
              n161 = in-place-array #11(w246, w245) -> (w251:T9)
              n162 = Bundle By Name(cluster=w251, "Marker Line Width"=w249) -> (w250:T9)
              n163 = in-place-array #11(w250) -> (w244:T8)  [unwired: 1 out]
            }
            n164 = call <vilib>:"Num to Bool Array.vi"("Array Size"=6, "Value"=w236) -> ("Bool Array"=w243:bool[])  [unwired: 9 out]
            n165 = Array To Cluster(array=w243) -> (cluster=w237:T18)
            n166 = local write "Marker Line Width"(w237) -> ()
            n167 = Bundle By Name(cluster=w248, "2D Error Bar Property Array"=w244) -> (w247:T5)
          }
          event "Marker Color": Value Change {
            n168 = event-data() -> ("NewVal"=w253:u32)  [unwired: 1 out]
            n169 = Unbundle By Name(w259) -> ("2D Error Bar Property Array"=w257:T8)
            n170 = local read "Active Plot"() -> (w256:i32)
            n171 = in-place {
              in-place-border: w253 -> [w260]
              n172 = in-place-array #12(w257, w256) -> (w262:T9)
              n173 = Bundle By Name(cluster=w262, "Marker Color"=w260) -> (w261:T9)
              n174 = in-place-array #12(w261) -> (w255:T8)  [unwired: 1 out]
            }
            n175 = Bundle By Name(cluster=w259, "2D Error Bar Property Array"=w255) -> (w258:T5)
          }
          event "Marker Size": Value Change {
            n176 = event-data() -> ("NewVal"=w264:dbl)  [unwired: 1 out]
            n177 = local read "Active Plot"() -> (w267:i32)
            n178 = Unbundle By Name(w270) -> ("2D Error Bar Property Array"=w268:T8)
            n179 = in-place {
              in-place-border: w264 -> [w271]
              n180 = in-place-array #13(w268, w267) -> (w273:T9)
              n181 = Bundle By Name(cluster=w273, "Marker Size"=w271) -> (w272:T9)
              n182 = in-place-array #13(w272) -> (w266:T8)  [unwired: 1 out]
            }
            n183 = Bundle By Name(cluster=w270, "2D Error Bar Property Array"=w266) -> (w269:T5)
          }
          event "Error Mode": Value Change {
            n184 = event-data() -> ("NewVal"=w275:u16)  [unwired: 1 out]
            n185 = Unbundle By Name(w282) -> ("2D Error Bar Property Array"=w280:T8)
            n186 = local read "Active Plot"() -> (w279:i32)
            n187 = case shown="1" w275 {
              tunnel: [T16."Show Y Error" ("Error Mode") T16."Show Both Error" ("Error Mode")] -> w274
              frame 0, Default {
              }
              frame 1 {
              }
            }
            n188 = in-place {
              in-place-border: w274 -> [w285]
              n189 = in-place-array #14(w280, w279) -> (w287:T9)
              n190 = Bundle By Name(cluster=w287, "Error Mode"=w285) -> (w286:T9)
              n191 = in-place-array #14(w286) -> (w278:T8)  [unwired: 1 out]
            }
            n192 = Bundle By Name(cluster=w282, "2D Error Bar Property Array"=w278) -> (w281:T5)
          }
          event User Event {
            n193 = event-data() -> ()  [unwired: 6 out]
          }
        }
        n194 = case shown="True" w71 {
          tunnel: w73 -> [_ w78]
          frame False {
          }
          frame True {
            n195 = call <vilib>:"Temp Graph Update.vi"("Property Name"=Temp_Graph_Property_Action."Plots Property", "State"=Temp_Graph_State."Update Graph", "Property In"=w78) -> ()  [unwired: 2 in, 7 out]
          }
        }
      }
      frame "Exit" {
      }
    }
  }
  "Error Bar Property Out" <- w1
